vi "DevB.Error handler.vi"(8 "error in (no error)":errorcluster, 11 "DevB Session in":T1) -> (0 "error out":errorcluster, 3 "DevB Session out":T1)   [LabVIEW 2018]
uses:
  typedefs/DevB.Message Session.ctl
  typedefs/DevB.Message.ctl
  typedefs/DevB.Message type.ctl
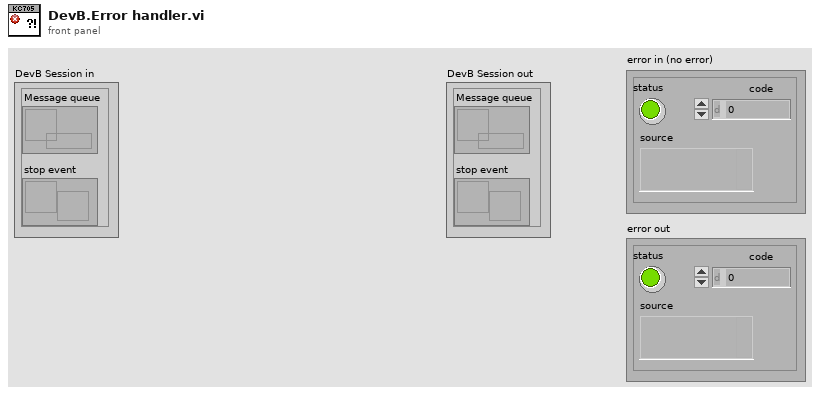
[diagram p1: front panel]
types:
  T1 = typedef "DevB.Message Session.ctl" = cluster{"Message queue":refnum<queue>, "stop event":refnum<user-event>}
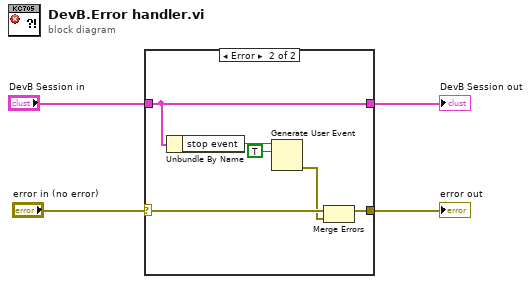
[diagram p0: block diagram]
diagram:
  n1 = case shown="Error" "error in (no error)" {
    selector: "error in (no error)" -> [w6 w9]
    tunnel: [w6 w8] -> w3
    tunnel: "DevB Session in" -> [w5 w10]
    tunnel: [w5 w10] -> w1
    frame No Error {
    }
    frame Error {
      n2 = Unbundle By Name(w10) -> ("stop event"=w12:refnum<user-event>)
      n3 = Generate User Event(user event=w12, event data cluster=TRUE ("event data")) -> (error out=w7:errorcluster)  [unwired: 2 in, 1 out]
      n4 = Merge Errors(w9, w7) -> (w8:errorcluster)
    }
  }
  "error out" <- w3
  "DevB Session out" <- w1
